vi "Write_Class_Multimeter.vi"(8 "error in (no error)":errorcluster caption="entrée d'erreur (pas d'erreur)", 10 "Class Spectrum Analyser":refnum<class "Class Spectrum Analyser (Default).lvclass">, 11 "Class Instrument Multimeter en entrée":refnum<class "Class Instrument Spectrum_Analyser.lvclass">) -> (0 "error out":errorcluster caption="sortie d'erreur", 3 "Class Instrument Multimeter en sortie":refnum<class "Class Instrument Spectrum_Analyser.lvclass">)   [LabVIEW 2020, in "Library Instrument & Equipement.lvlib" / "Library Instruments.lvlib" / "Class Instrument Spectrum_Analyser.lvclass"]
uses:
  Class Instrument Spectrum_Analyser.lvclass
  Spectrum Analyser/Class Spectrum Analyser (Default)/Class Spectrum Analyser (Default).lvclass
  Class Instrument Spectrum_Analyser.lvclass/Class Instrument Spectrum_Analyser.ctl
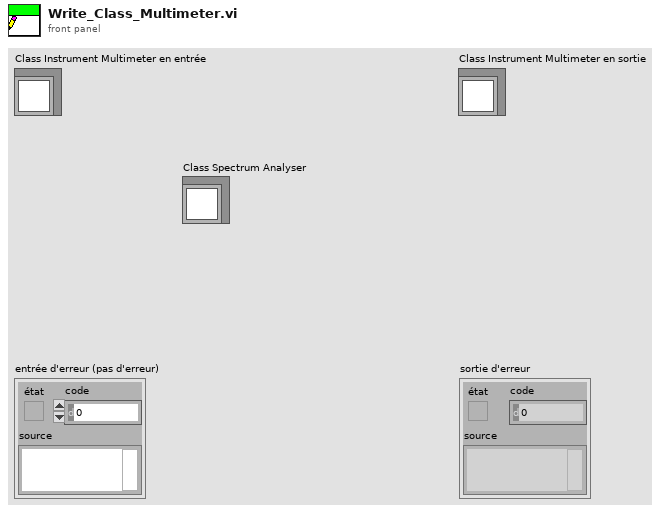
[diagram p1: front panel]
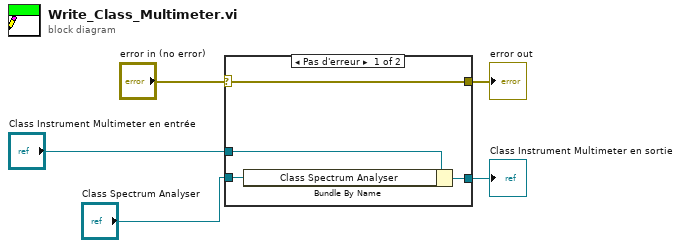
[diagram p0: block diagram]
diagram:
  n1 = case shown="Pas d'erreur" "error in (no error)" {
    selector: "error in (no error)" -> [w9 w10]
    tunnel: [w9 w10] -> w4
    tunnel: [w7 w11] -> w2
    tunnel: "Class Instrument Multimeter en entrée" -> [w8 w11]
    tunnel: "Class Spectrum Analyser" -> [w6 _]
    frame No Error {
      n2 = Bundle By Name(cluster=w8, "Class Spectrum Analyser"=w6) -> (w7:refnum<class "Class Instrument Spectrum_Analyser.lvclass">)
    }
    frame Error {
    }
  }
  "error out" <- w4
  "Class Instrument Multimeter en sortie" <- w2
